vi "open_ophir_device.vi"(8 "error in (no error)":errorcluster, 11 "OphirLMMeasurementLib.ICoLMMeasurement":refnum<k7>) -> (0 "error out":errorcluster, 1 "hDevice":i32, 2 "Device Serial Number":string, 3 "Orphir COM":refnum<k7>, 5 "data":variant)   [LabVIEW 2020]
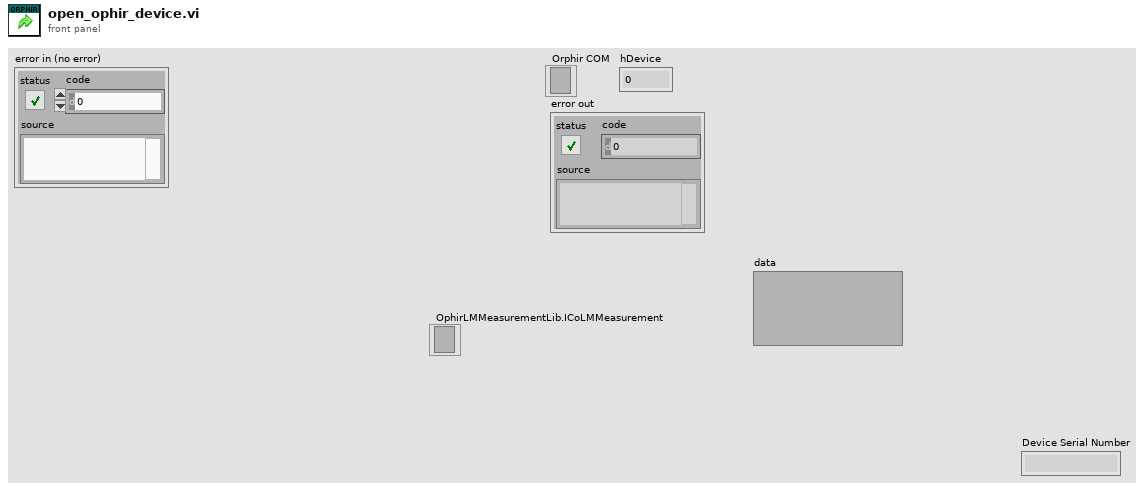
[diagram p1: front panel]
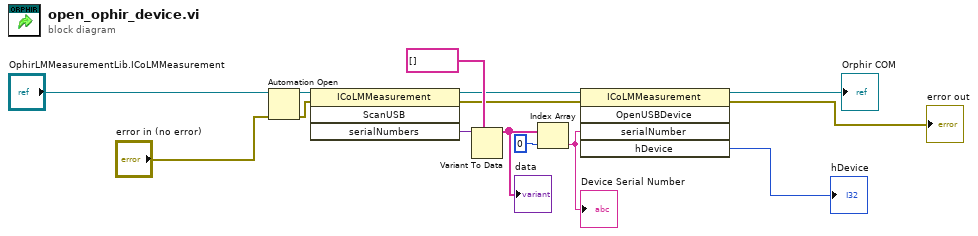
[diagram p0: block diagram]
diagram:
  n1 = Automation Open(error in (no error)="error in (no error)", Automation Refnum="OphirLMMeasurementLib.ICoLMMeasurement") -> (Automation Refnum=w13:refnum<k7>, error out=w4:errorcluster)  [unwired: 2 in]
  n2 = invoke class="ICoLMMeasurement" method="ScanUSB"(reference=w13, error in=w4) -> (reference out=w7:refnum<k7>, error out=w5:errorcluster, "serialNumbers"=w12:variant)  [unwired: 2 in, 1 out]
  n3 = Variant To Data(type=string[] [], Variant=w12) -> (data=w10:string[])  [unwired: 1 in, 1 out]
  "data" <- w10
  n4 = Index Array(array=w10, index=0) -> (element=w8:string)
  "Device Serial Number" <- w8
  n5 = invoke class="ICoLMMeasurement" method="OpenUSBDevice"(reference=w7, error in=w5, "serialNumber"=w8) -> (reference out=→"Orphir COM":refnum<k7>, error out=→"error out":errorcluster, "hDevice"=→"hDevice":i32)  [unwired: 2 in, 2 out]
